vi "AnalyzePulseTrain.vi"(0 "Waveform In":waveform(dbl)={"t0"=timestamp(3433165898.5470004 s since 1904-01-01), "dt"=1e-05, "Y"=array[4250 elements]}, 5 "Repetitions in the Input Waveform":i32, 7 "Pulse Characteristics":T2={"Pulses per Cycle"=2, "Load Resistance (Ohms)"=750.0, "Krec Value"=2, "Recovery Mode (T=Active)"=TRUE, "Target Stim Currents (Amps)"=[]}) -> (2 "Avg. CBC Width":dbl format="%0.2f", 3 "Avg. CBC Amplitude":dbl format="%0.2f", 4 "Stim PW":dbl[](array[numeric]), 6 "Stim Amplitude":dbl[](array[numeric]), 8 "Interphase Delay":dbl[](array[numeric]), 10 "Recovery PW":dbl[](array[numeric]), 12 "Waveform Parameters":T1, 13 "Frequency":dbl, 14 "Recovery Holdoff":dbl[](array[numeric]), 15 "Recovery Amplitude":dbl[](array[numeric]))   [LabVIEW 2010]
uses:
  <vilib>/measure/mamon.llb/Trigger Detection for 1 Channel.vi
  <vilib>/measure/NI_MAPro.lvlib
  <vilib>/Analysis/NI_AALBase.lvlib
panel:
  out "Normalized Waveform":waveform(dbl)(graph)
  # "The input waveform should be a capture of the STIM chip output\n(before the cap) when the output is held at 1/2 HVDD by the\nLoad Resistance.  This ensures that passive recovery and CBC\npulses are captured, because they look like pulses pulled to GND."
  # "The elements in these arrays correspond to the pulses per cycle.\nThey are the averages over all the repetitions in the waveform."
  # "Enter Target Current\nfor each in array below"
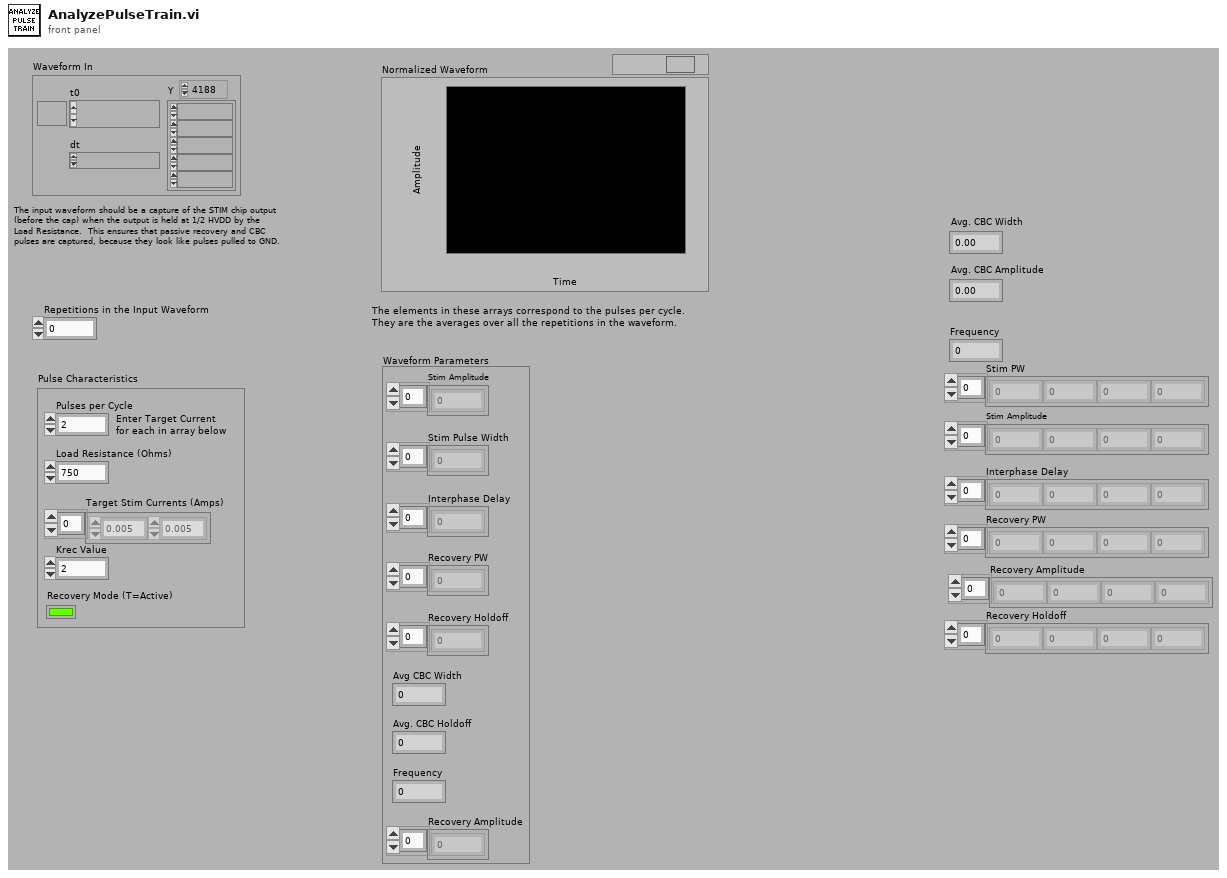
[diagram p1: front panel]
types:
  T1 = cluster{"Stim Amplitude":dbl[], "Stim Pulse Width":dbl[], "Interphase Delay":dbl[], "Recovery PW":dbl[], "Recovery Holdoff":dbl[], "Avg CBC Width":dbl, "Frequency":dbl, "Avg. CBC Holdoff":dbl, "Recovery Amplitude":dbl[]}
  T2 = cluster{"Pulses per Cycle":i32, "Load Resistance (Ohms)":dbl, "Krec Value":i32, "Recovery Mode (T=Active)":bool, "Target Stim Currents (Amps)":dbl[]}
  T3 = cluster{"trigger slope":u16, "Trigger Level":dbl}[]
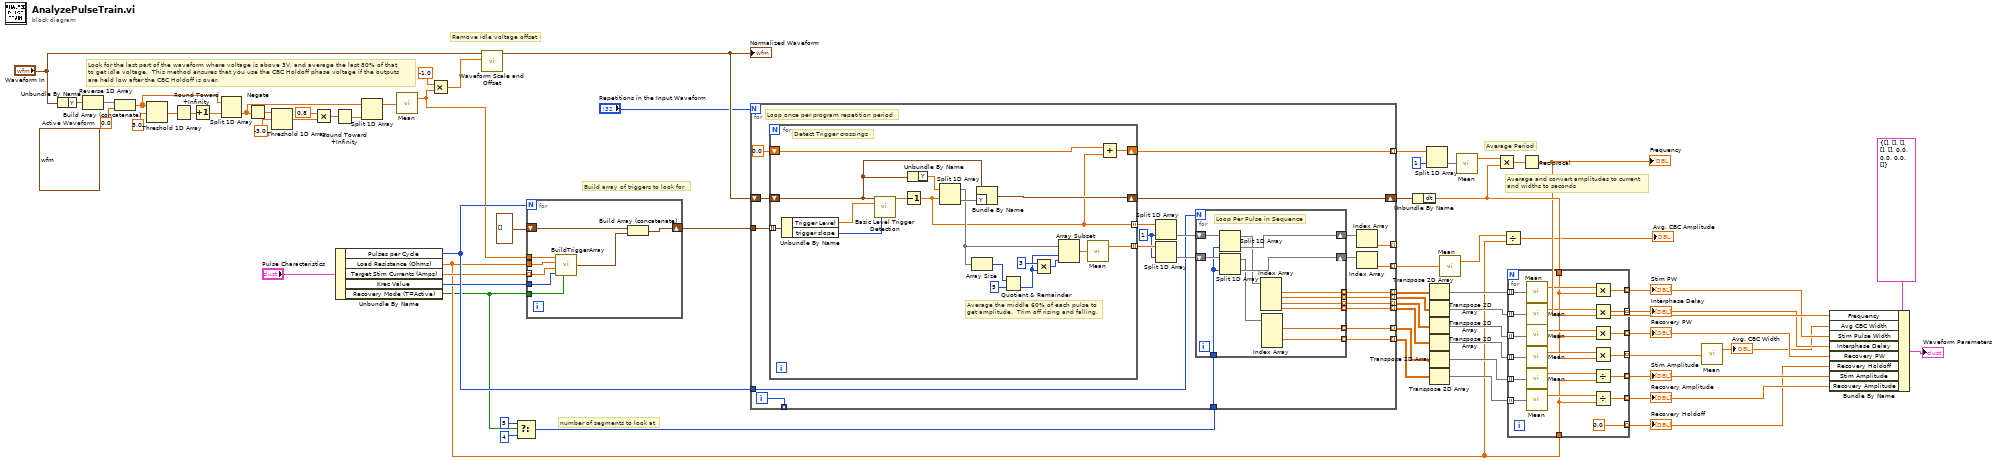
[diagram p0: block diagram]
diagram:
  (unwired) waveform(dbl) {"t0"=timestamp(3418839276.250478 s since 1904-01-01), "dt"=1e-06, "Y"=[5.0, 5.0, 9.0, 9.0, 9.0, 9.0, 9.0, 9.0, 9.0, 9.0, 5.0, 5.0, 5.0, 3.0, 3.0, 3.0, 3.0, 3.0, 3.0, 3.0, 3.0, 3.0, 3.0, 3.0, 3.0, 3.0, 3.0, 3.0, 3.0, 5.0, 5.0, 5.0, 5.0, 8.0, 8.0, 8.0, 8.0, 8.0, 8.0, 8.0, 8.0, 5.0, 5.0, 5.0, 3.0, 3.0, 3.0, 3.0, 3.0, 3.0, 3.0, 3.0, 3.0, 3.0, 3.0, 3.0, 3.0, 3.0, 3.0, 3.0, 5.0, 5.0, 5.0, 5.0, 0.0, 0.0, 0.0, 0.0, 0.0, 5.0, 5.0, 5.0, 5.0, 5.0, 5.0, 5.0, 5.0, 5.0, 5.0, 5.0, 5.0, 5.0, 5.0, 5.0, 5.0, 5.0, 5.0, 5.0, 5.0, 5.0, 5.0, 5.0, 5.0, 5.0, 5.0, 5.0, 5.0, 5.0, 5.0, 5.0, 5.0, 5.0, 9.0, 9.0, 9.0, 9.0, 9.0, 9.0, 9.0, 9.0, 5.0, 5.0, 5.0, 3.0, 3.0, 3.0, 3.0, 3.0, 3.0, 3.0, 3.0, 3.0, 3.0, 3.0, 3.0, 3.0, 3.0, 3.0, 3.0, 5.0, 5.0, 5.0, 5.0, 8.0, 8.0, 8.0, 8.0, 8.0, 8.0, 8.0, 8.0, 5.0, 5.0, 5.0, 3.0, 3.0, 3.0, 3.0, 3.0, 3.0, 3.0, 3.0, 3.0, 3.0, 3.0, 3.0, 3.0, 3.0, 3.0, 3.0, 5.0, 5.0, 5.0, 5.0, 0.0, 0.0, 0.0, 0.0, 0.0, 5.0, 5.0, 5.0, 5.0, 5.0, 5.0, 5.0, 5.0, 5.0, 5.0, 5.0, 5.0, 5.0, 5.0, 5.0, 5.0, 5.0, 5.0, 5.0, 5.0, 5.0, 5.0, 5.0, 5.0, 5.0, 5.0, 5.0, 5.0, 5.0, 5.0, 5.0, 5.0, 5.0, 9.0, 9.0, 9.0, 9.0, 9.0, 9.0, 9.0, 9.0, 5.0, 5.0, 5.0, 3.0, 3.0, 3.0, 3.0, 3.0, 3.0, 3.0, 3.0, 3.0, 3.0, 3.0, 3.0, 3.0, 3.0, 3.0, 3.0, 5.0, 5.0, 5.0, 5.0, 8.0, 8.0, 8.0, 8.0, 8.0, 8.0, 8.0, 8.0, 5.0, 5.0, 5.0, 3.0, 3.0, 3.0, 3.0, 3.0, 3.0, 3.0, 3.0, 3.0, 3.0, 3.0, 3.0, 3.0, 3.0, 3.0, 3.0, 5.0, 5.0, 5.0, 5.0, 0.0, 0.0, 0.0, 0.0, 0.0, 5.0, 5.0, 5.0, 5.0, 5.0, 5.0, 5.0, 5.0, 5.0, 5.0, 5.0, 5.0, 5.0, 5.0, 5.0, 5.0, 5.0, 5.0, 5.0, 5.0, 5.0, 5.0, 5.0, 5.0, 5.0, 5.0, 5.0, 5.0, 5.0, 5.0, 5.0, 5.0, 5.0, 9.0, 9.0, 9.0, 9.0, 9.0, 9.0, 9.0, 9.0, 5.0, 5.0, 5.0, 3.0, 3.0, 3.0, 3.0, 3.0, 3.0, 3.0, 3.0, 3.0, 3.0, 3.0, 3.0, 3.0, 3.0, 3.0, 3.0, 5.0, 5.0, 5.0, 5.0, 8.0, 8.0, 8.0, 8.0, 8.0, 8.0, 8.0, 8.0, 5.0, 5.0, 5.0, 3.0, 3.0, 3.0, 3.0, 3.0, 3.0, 3.0, 3.0, 3.0, 3.0, 3.0, 3.0, 3.0, 3.0, 3.0, 3.0, 5.0, 5.0, 5.0, 5.0, 0.0, 0.0, 0.0, 0.0, 0.0, 5.0, 5.0, 5.0, 5.0, 5.0, 5.0, 5.0, 5.0, 5.0, 5.0, 5.0, 5.0, 5.0, 5.0, 5.0, 5.0, 5.0, 5.0, 5.0, 5.0, 5.0, 5.0, 5.0, 5.0, 5.0, 5.0, 5.0, 5.0, 5.0, 5.0, 5.0, 5.0, 5.0, 9.0, 9.0, 9.0, 9.0, 9.0, 9.0, 9.0, 9.0, 5.0, 5.0, 5.0, 3.0, 3.0, 3.0, 3.0, 3.0, 3.0, 3.0, 3.0, 3.0, 3.0, 3.0, 3.0, 3.0, 3.0, 3.0, 3.0, 5.0, 5.0, 5.0, 5.0, 8.0, 8.0, 8.0, 8.0, 8.0, 8.0, 8.0, 8.0, 5.0, 5.0, 5.0, 3.0, 3.0, 3.0, 3.0, 3.0, 3.0, 3.0, 3.0, 3.0, 3.0, 3.0, 3.0, 3.0, 3.0, 3.0, 3.0, 5.0, 5.0, 5.0, 5.0, 0.0, 0.0, 0.0, 0.0, 0.0, 5.0, 5.0, 5.0, 5.0, 5.0, 5.0, 5.0, 5.0, 5.0, 5.0, 5.0, 5.0, 5.0, 5.0, 5.0, 5.0, 5.0, 5.0, 5.0, 5.0, 5.0, 5.0, 5.0, 5.0, 5.0, 5.0, 5.0, 5.0, 5.0, 5.0, 5.0, 5.0, 5.0, 5.0]}  # Active Waveform
  # "number of segments to look at"
  # "Look for the last part of the waveform where voltage is above 3V, and average the last 80% of that\nto get idle voltage.  This method ensures that you use the CBC Holdoff phase voltage if the outputs\nare held low after the CBC Holdoff is over."
  # "Average Period"
  # "Average and convert amplitudes to current\nand widths to seconds"
  # "Build array of triggers to look for"
  # "Remove idle voltage offset"
  n1 = Unbundle By Name("Waveform In") -> ("Y"=w25:dbl[])
  n2 = Reverse 1D Array(array=w25) -> (reversed array=w24:dbl[])
  n3 = Build Array (concatenate)(w24, 0.0 ("y")) -> (w19:dbl[])
  n4 = Threshold 1D Array(2:3.0 ("y"), 3:w19) -> (0:w21:dbl)  [unwired: 1 in]
  n5 = Round Toward +Infinity(x=w21) -> (ceil(x): smallest int >= x=w20:dbl)
  n6 = Increment(x=w20) -> (x+1=w10:dbl)
  n7 = Split 1D Array(array=w19, index=w10) -> (second subarray=w12:dbl[])  [unwired: 1 out]
  n8 = Negate(x=w12) -> (-x=w17:dbl[])
  n9 = Threshold 1D Array(2:-3.0 ("y"), 3:w17) -> (0:w16:dbl)  [unwired: 1 in]
  n10 = Multiply(x=0.8, y=w16) -> (x*y=w14:dbl)
  n11 = Round Toward +Infinity(x=w14) -> (ceil(x): smallest int >= x=w13:dbl)
  n12 = Unbundle By Name("Pulse Characteristics") -> ("Pulses per Cycle"=w47:i32, "Load Resistance (Ohms)"=w41:dbl, "Target Stim Currents (Amps)"=w46:dbl[], "Krec Value"=w45:i32, "Recovery Mode (T=Active)"=w4:bool)
  n13 = Split 1D Array(array=w12, index=w13) -> (first subarray=w11:dbl[])  [unwired: 1 out]
  n14 = call <vilib>:"Mean.vi"("X"=w11) -> ("mean"=w5:dbl)  [unwired: 1 out]
  n15 = Multiply(x=-1.0, y=w5) -> (x*y=w62:dbl)
  n16 = call <vilib>:"Waveform Scale and Offset.vi"("offset"=w62, "waveform in"="Waveform In") -> ("waveform out"=w61:waveform(dbl))  [unwired: 8 in, 1 out]
  "Normalized Waveform" <- w61
  n17 = Select(t=5, s=w4, f=4 ("index")) -> (s? t:f=w2:i32)
  n18 = for {
    N: w47 -> [_]
    shift-right: [w74] -> w9
    shift-left: T3 [] -> [w73]
    tunnel: w5 -> [w72]
    tunnel: w4 -> [w71]
    tunnel: w41 -> [w70]
    tunnel: w46 -> [w69] mode=indexing
    tunnel: w45 -> [w68]
    n19 = call "BuildTriggerArray.vi"("CBC Trigger Level"=w72, "Load Resistance (Ohms)"=w70, "Target Stim Current (Amps)"=w69, "Krec Value"=w68, "Recovery Mode (T=Active)"=w71) -> ("Pulse Triggers"=w67:T3)
    n20 = Build Array (concatenate)(w73, w67) -> (w74:T3)
  }
  n21 = for {
    N: "Repetitions in the Input Waveform" -> [_]
    tunnel: w9 -> [w97]
    shift-right: [w93] -> w43
    shift-left: w61 -> [w96]
    tunnel: w47 -> [w90]
    tunnel: [w87] -> _ mode=indexing
    tunnel: [w86] -> w60 mode=indexing
    tunnel: [w85] -> w59 mode=indexing
    tunnel: [w84] -> w58 mode=indexing
    tunnel: [w83] -> w57 mode=indexing
    tunnel: [w82] -> w56 mode=indexing
    tunnel: [w81] -> w55 mode=indexing
    tunnel: [w80] -> w54 mode=indexing
    tunnel: [w77] -> w40 mode=indexing
    tunnel: w2 -> [w76]
    tunnel: [w75] -> _ mode=indexing
    i -> [w75]
    w94 = 1 ("index")
    # "Loop once per program repetition period"
    n22 = for {
      tunnel: w97 -> [w129] mode=indexing
      shift-right: [w115] -> w93
      shift-left: w96 -> [w124]
      tunnel: [w116] -> w95 mode=indexing
      tunnel: [w111] -> w78 mode=indexing
      shift-right: [w114] -> w77
      shift-left: 0.0 -> [w113]
      # "Detect Trigger crossings"
      # "Average the middle 60% of each pulse to\nget amplitude.  Trim off rising and falling."
      n23 = Unbundle By Name(w129) -> ("Trigger Level"=w128:dbl, "trigger slope"=w127:u16)
      n24 = call-poly <vilib>:"Basic Level Trigger Detection.vi"("signal in"=w124, "level"=w128, "trigger slope"=w127) -> ("trigger location"=w112:dbl)  [unwired: 10 in, 2 out]
      n25 = Decrement(x=w112) -> (x-1=w111:dbl)
      n26 = Unbundle By Name(w124) -> ("Y"=w126:dbl[])
      n27 = Split 1D Array(array=w126, index=w111) -> (first subarray=w118:dbl[], second subarray=w125:dbl[])
      n28 = Array Size(array=w118) -> (size(s)=w123:i32)
      n29 = Bundle By Name(cluster=w124, "Y"=w125) -> (w115:waveform(dbl))
      n30 = Quotient & Remainder(x=w123, y=5) -> (floor(x/y)=w120:i32)  [unwired: 1 out]
      n31 = Multiply(x=3, y=w120) -> (x*y=w119:i32)
      n32 = Array Subset(array=w118, index=w120, length=w119) -> (w117:dbl[])
      n33 = call <vilib>:"Mean.vi"("X"=w117) -> ("mean"=w116:dbl)  [unwired: 1 out]
      n34 = Add(x=w113, y=w111) -> (x+y=w114:dbl)
    }
    n35 = Split 1D Array(array=w78, index=w94) -> (second subarray=w92:dbl[])  [unwired: 1 out]
    n36 = Split 1D Array(array=w95, index=w94) -> (second subarray=w91:dbl[])  [unwired: 1 out]
    n37 = for {
      N: w90 -> [_]
      shift-right: [w108] -> w89
      shift-left: w92 -> [w110]
      shift-right: [w107] -> w88
      shift-left: w91 -> [w109]
      tunnel: [w104] -> w85 mode=indexing
      tunnel: [w103] -> w84 mode=indexing
      tunnel: [w102] -> w83 mode=indexing
      tunnel: [w101] -> w82 mode=indexing
      tunnel: [w100] -> w81 mode=indexing
      tunnel: [w99] -> w80 mode=indexing
      tunnel: w76 -> [w98]
      # "Loop Per Pulse in Sequence"
      n38 = Split 1D Array(array=w110, index=w98) -> (first subarray=w106:dbl[], second subarray=w108:dbl[])
      n39 = Split 1D Array(array=w109, index=w98) -> (first subarray=w105:dbl[], second subarray=w107:dbl[])
      n40 = Index Array(array=w106) -> (element #1=w104:dbl, element #2=w103:dbl, element #3=w102:dbl, element #4=w101:dbl)  [unwired: 4 in]
      n41 = Index Array(array=w105) -> (element #1=w100:dbl, element #3=w99:dbl)  [unwired: 4 in, 2 out]
    }
    n42 = Index Array(array=w89) -> (element=w87:dbl)  [unwired: 1 in]
    n43 = Index Array(array=w88) -> (element=w86:dbl)  [unwired: 1 in]
  }
  n44 = Unbundle By Name(w43) -> ("dt"=w37:dbl)
  n45 = Split 1D Array(array=w40, index=1) -> (second subarray=w39:dbl[])  [unwired: 1 out]
  n46 = Transpose 2D Array(2D array=w59) -> (transposed array=w53:dbl[][])
  n47 = Transpose 2D Array(2D array=w58) -> (transposed array=w52:dbl[][])
  n48 = Transpose 2D Array(2D array=w57) -> (transposed array=w51:dbl[][])
  n49 = Transpose 2D Array(2D array=w56) -> (transposed array=w50:dbl[][])
  n50 = Transpose 2D Array(2D array=w55) -> (transposed array=w49:dbl[][])
  n51 = Transpose 2D Array(2D array=w54) -> (transposed array=w48:dbl[][])
  n52 = call <vilib>:"Mean.vi"("X"=w60) -> ("mean"=w42:dbl)  [unwired: 1 out]
  n53 = call <vilib>:"Mean.vi"("X"=w39) -> ("mean"=w38:dbl)  [unwired: 1 out]
  n54 = Multiply(x=w38, y=w37) -> (x*y=w36:dbl)
  n55 = Divide(x=w42, y=w41) -> (x/y=→"Avg. CBC Amplitude":dbl)
  n56 = for {
    tunnel: w53 -> [w150] mode=indexing
    tunnel: w52 -> [w149] mode=indexing
    tunnel: w51 -> [w148] mode=indexing
    tunnel: w50 -> [w147] mode=indexing
    tunnel: w49 -> [w146] mode=indexing
    tunnel: w48 -> [w145] mode=indexing
    tunnel: [w144] -> w31 mode=indexing
    tunnel: [w143] -> w30 mode=indexing
    tunnel: [w142] -> w29 mode=indexing
    tunnel: [w141] -> w7 mode=indexing
    tunnel: [w140] -> w28 mode=indexing
    tunnel: [w139] -> w27 mode=indexing
    tunnel: w37 -> [w132]
    tunnel: w41 -> [w131]
    tunnel: [0.0 ("Load Resistance (Ohms)")] -> w8 mode=indexing
    n57 = call <vilib>:"Mean.vi"("X"=w150) -> ("mean"=w137:dbl)  [unwired: 1 out]
    n58 = call <vilib>:"Mean.vi"("X"=w149) -> ("mean"=w136:dbl)  [unwired: 1 out]
    n59 = call <vilib>:"Mean.vi"("X"=w148) -> ("mean"=w135:dbl)  [unwired: 1 out]
    n60 = call <vilib>:"Mean.vi"("X"=w147) -> ("mean"=w134:dbl)  [unwired: 1 out]
    n61 = call <vilib>:"Mean.vi"("X"=w146) -> ("mean"=w133:dbl)  [unwired: 1 out]
    n62 = call <vilib>:"Mean.vi"("X"=w145) -> ("mean"=w138:dbl)  [unwired: 1 out]
    n63 = Multiply(x=w137, y=w132) -> (x*y=w144:dbl)
    n64 = Multiply(x=w136, y=w132) -> (x*y=w143:dbl)
    n65 = Multiply(x=w135, y=w132) -> (x*y=w142:dbl)
    n66 = Multiply(x=w134, y=w132) -> (x*y=w141:dbl)
    n67 = Divide(x=w133, y=w131) -> (x/y=w140:dbl)
    n68 = Divide(x=w138, y=w131) -> (x/y=w139:dbl)
  }
  "Stim PW" <- w31
  "Interphase Delay" <- w30
  "Recovery PW" <- w29
  "Recovery Holdoff" <- w8
  "Stim Amplitude" <- w28
  "Recovery Amplitude" <- w27
  n69 = Reciprocal(x=w36) -> (1/x=w33:dbl)
  "Frequency" <- w33
  n70 = call <vilib>:"Mean.vi"("X"=w7) -> ("mean"=w6:dbl)  [unwired: 1 out]
  "Avg. CBC Width" <- w6
  n71 = Bundle By Name(cluster=T1 {"Stim Amplitude"=[], "Stim Pulse Width"=[], "Interphase Delay"=[], "Recovery PW"=[], "Recovery Holdoff"=[], "Avg CBC Width"=0.0, "Frequency"=0.0, "Avg. CBC Holdoff"=0.0, "Recovery Amplitude"=[]} ("Pulse Train Parameters"), "Frequency"=w33, "Avg CBC Width"=w6, "Stim Pulse Width"=w31, "Interphase Delay"=w30, "Recovery PW"=w29, "Recovery Holdoff"=w8, "Stim Amplitude"=w28, "Recovery Amplitude"=w27) -> (→"Waveform Parameters":T1)
